vi "Lidar Subsystem.vi"() -> ()   [LabVIEW 2009]
uses:
  <vilib>/rvi/FXPMathLib/FxpSinAndCos/XNode/nifxpmath_SinAndCos.xnode
  <vilib>/rvi/FXPMathLib/FxpSinAndCos/simVIs/DllFxpSinAndCosTemp_sub.vi
  <vilib>/rvi/FXPMathLib/FxpSinAndCos/subVIs/nifxpmath_SinAndCos_SimConfig.ctl
  <vilib>/rvi/FXPMathLib/FxpAdd/XNode/nifxpmath_Add.xnode
  <vilib>/rvi/FXPMathLib/FxpAdd/simVIs/DllFxpAddTemp_sub.vi
  <vilib>/fxp/LVFixedPointOverflowPolicyTypeDef.ctl
  <vilib>/fxp/LVFixedPointQuantizationPolicyTypeDef.ctl
  <vilib>/rvi/FXPMathLib/FxpAdd/subVIs/nifxpmath_Add_SimConfig.ctl
  Motor Control Global.vi
  <vilib>/rvi/FXPMathLib/FxpMul/XNode/nifxpmath_Multiplier.xnode
  <vilib>/rvi/FXPMathLib/FxpMul/simVIs/DllFxpMulTemp_sub.vi
  <vilib>/rvi/FXPMathLib/FxpMul/subVIs/nifxpmath_Mul_SimConfig.ctl
panel:
  in  "frequency, in pi rad/cycle":fxp<+/-,16,1> format="%.16g"
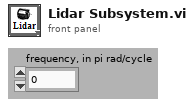
[diagram p1: front panel]
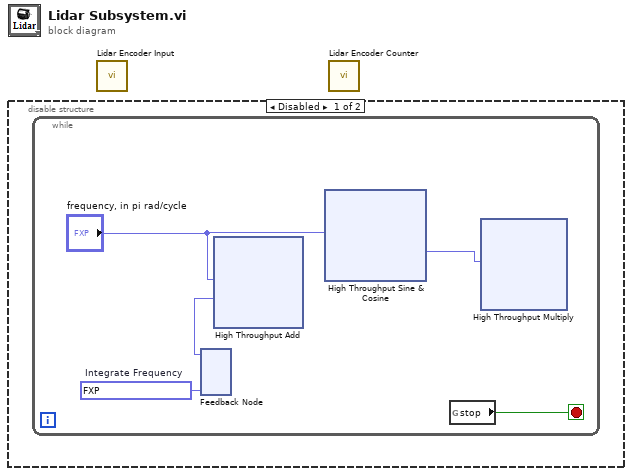
[diagram p0: block diagram]
diagram:
  n1 = disable-structure shown="Disabled" {
    frame #0 {
      n2 = while {
        stop <- w2 stop-if-true
        w3 = fxp<+/-,16,1> 0.0  # Integrate Frequency
        n3 = feedback #1(w3) -> (w6:fxp<+/-,16,1>)
        n4 = xnode "High Throughput Add"("x"="frequency, in pi rad/cycle", "y"=w6) -> ("x+y"=w5:fxp<+/-,16,1>)
        n5 = xnode "High Throughput Sine & Cosine"("x (pi)"="frequency, in pi rad/cycle") -> ("sin(x)"=w1:fxp<+/-,16,2>)  [unwired: 1 out]
        n6 = global read "Motor Control Global.vi" "stop"() -> (w2:bool)
        n7 = xnode "High Throughput Multiply"("x"=w1) -> ()  [unwired: 1 in, 1 out]
      }
    }
    frame #1 {
    }
  }
  n8 = call "Lidar Encoder Input.vi"() -> ()  [unwired: 1 in]
  n9 = call "Lidar Encoder Counter.vi"() -> ()  [unwired: 1 in]
